vi "LC_PV_Act_Ctrl.vi"   [LabVIEW 2016]
doc: "-----------------------------------------------------------------------------------------------------------------------\nCopyright <2019> <The University of Tennessee at Knoxville and the University of Tennessee Research Foundation>\nThis software is released under BSD-3\nhttps://opensource.org/licenses/BSD-3-Clause \nAdditional license options available at https://utrf.tennessee.edu/industry/sample-agreements/\n-----------------------------------------------------------------------------------------------------------------------\n\n\nActive power support for PV local controller"
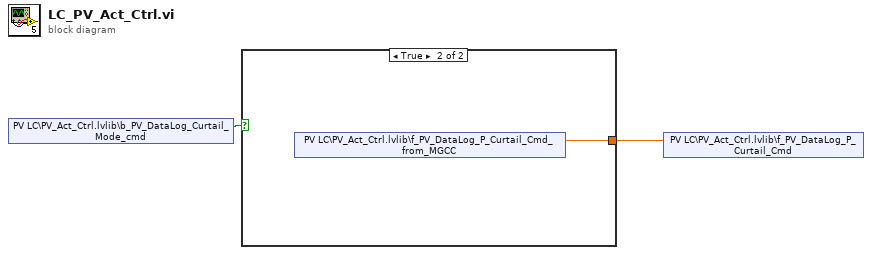
[diagram p0: block diagram]
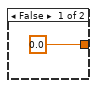
[diagram p2: hidden frame]
diagram:
  n1 = shared-variable "PV LC\\PV_Act_Ctrl.lvlib\\b_PV_DataLog_Curtail_Mode_cmd"() -> (w2:bool)  [unwired: 1 in, 1 out]
  n2 = case shown="True" w2 {
    tunnel: [0.0 ("f_PV_DataLog_P_Curtail_Cmd") w4] -> w1
    frame False {
    }
    frame True {
      n3 = shared-variable "PV LC\\PV_Act_Ctrl.lvlib\\f_PV_DataLog_P_Curtail_Cmd_from_MGCC"() -> (w4:dbl)  [unwired: 1 in, 1 out]
    }
  }
  n4 = shared-variable "PV LC\\PV_Act_Ctrl.lvlib\\f_PV_DataLog_P_Curtail_Cmd"(w1) -> ()  [unwired: 1 in, 1 out]
